vi "副屏设置.vi"() -> ()   [LabVIEW 2016, in "副屏.lvlib"]
uses:
  <vilib>/Utility/config.llb/NI_LVConfig.lvlib
panel:
  in  "藻密度":bool=TRUE caption="氨氮禁用"
  in  "叶绿素a":bool=TRUE caption="氨氮禁用"
  in  "启用副屏":bool=TRUE caption="氨氮禁用"
  in  "关闭":bool
  in  "底部状态栏显示信息":string="一体化微型水质监测系统"
  in  "流速":bool caption="氨氮禁用"
  in  "瞬时流量":bool caption="氨氮禁用"
  in  "湿度":bool=TRUE caption="氨氮禁用"
  in  "水位":bool caption="氨氮禁用"
  in  "室温":bool=TRUE caption="氨氮禁用"
  in  "CODCr":bool caption="氨氮禁用"
  in  "CODMn":bool caption="氨氮禁用"
  in  "总氮":bool caption="氨氮禁用"
  in  "总磷":bool caption="氨氮禁用"
  in  "氨氮":bool caption="氨氮禁用"
  in  "Turb":bool caption="氨氮禁用"
  in  "Cond":bool caption="氨氮禁用"
  in  "DO":bool caption="氨氮禁用"
  in  "pH":bool caption="氨氮禁用"
  in  "水温":bool caption="氨氮禁用"
  # "副屏显示信息设置"
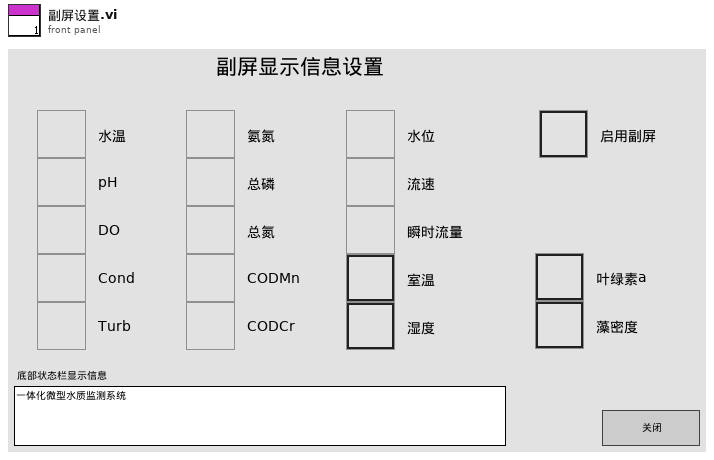
[diagram p1: front panel]
types:
  T1 = typedef "NI_LVConfig.lvlib/Config Data RefNum.ctl" = refnum<k1>
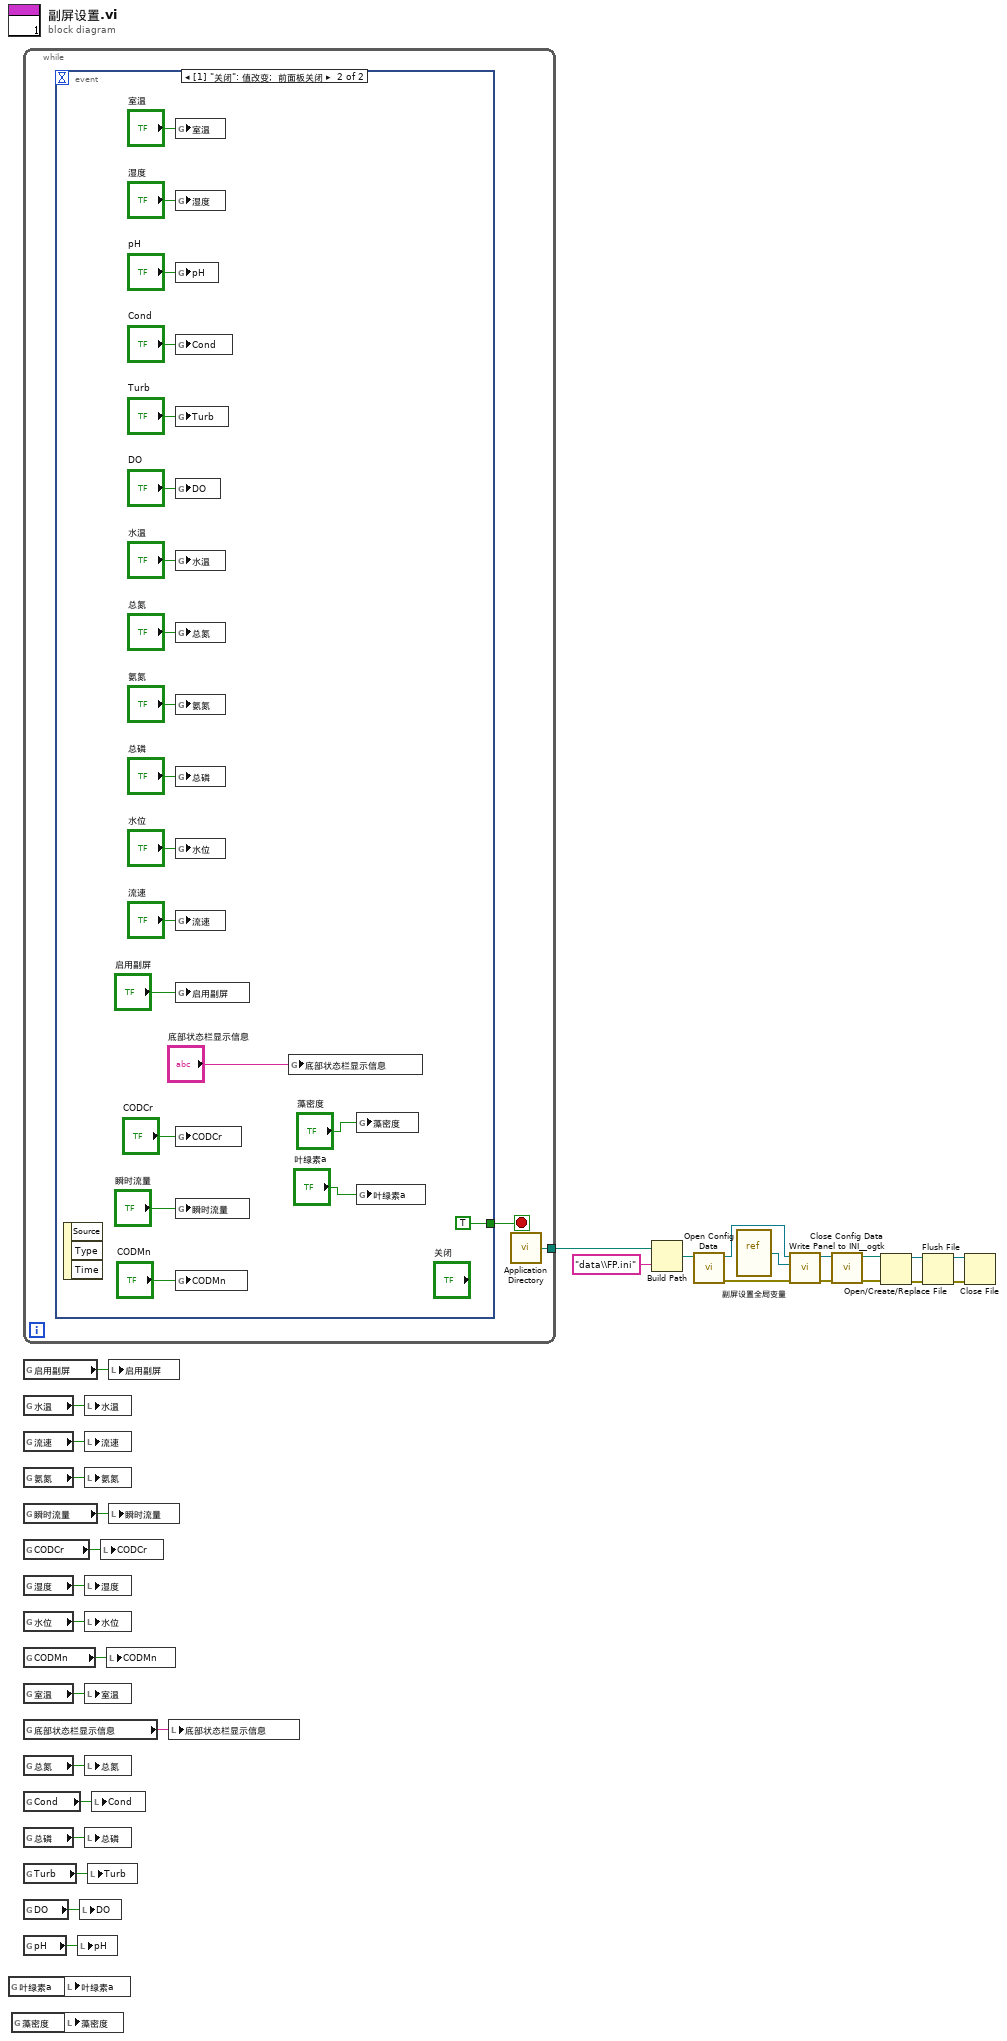
[diagram p0: block diagram]
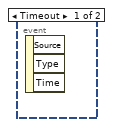
[diagram p2: hidden frame]
diagram:
  n1 = global read "副屏设置全局变量.vi" "叶绿素a"() -> (w7:bool)
  n2 = global read "副屏设置全局变量.vi" "藻密度"() -> (w8:bool)
  n3 = while {
    tunnel: [w34] -> w10
    stop <- w35 stop-if-true
    n4 = event shown="[1] \"关闭\": 值改变;  前面板关闭" {
      selector: _ -> [_ _]
      dyn-events: _ -> [_ _]
      timeout: _ -> [_ _]
      tunnel: [_ TRUE] -> w35
      event Timeout {
        n5 = event-data() -> ()  [unwired: 1 in, 3 out]
      }
      event "关闭": Value Change; Panel Close {
        n6 = event-data() -> ()  [unwired: 1 in, 3 out]
        n7 = global write "副屏设置全局变量.vi" "室温"("室温") -> ()
        n8 = global write "副屏设置全局变量.vi" "湿度"("湿度") -> ()
        n9 = global write "副屏设置全局变量.vi" "pH"("pH") -> ()
        n10 = global write "副屏设置全局变量.vi" "Cond"("Cond") -> ()
        n11 = global write "副屏设置全局变量.vi" "Turb"("Turb") -> ()
        n12 = global write "副屏设置全局变量.vi" "DO"("DO") -> ()
        n13 = global write "副屏设置全局变量.vi" "水温"("水温") -> ()
        n14 = global write "副屏设置全局变量.vi" "总氮"("总氮") -> ()
        n15 = global write "副屏设置全局变量.vi" "氨氮"("氨氮") -> ()
        n16 = global write "副屏设置全局变量.vi" "总磷"("总磷") -> ()
        n17 = global write "副屏设置全局变量.vi" "水位"("水位") -> ()
        n18 = global write "副屏设置全局变量.vi" "流速"("流速") -> ()
        n19 = global write "副屏设置全局变量.vi" "启用副屏"("启用副屏") -> ()
        n20 = global write "副屏设置全局变量.vi" "CODCr"("CODCr") -> ()
        n21 = global write "副屏设置全局变量.vi" "瞬时流量"("瞬时流量") -> ()
        n22 = global write "副屏设置全局变量.vi" "CODMn"("CODMn") -> ()
        n23 = global write "副屏设置全局变量.vi" "底部状态栏显示信息"("底部状态栏显示信息") -> ()
        n24 = global write "副屏设置全局变量.vi" "藻密度"("藻密度") -> ()
        n25 = global write "副屏设置全局变量.vi" "叶绿素a"("叶绿素a") -> ()
      }
    }
    n26 = call <vilib>:"Application Directory.vi"() -> ("Application Directory"=w34:path)
  }
  n27 = global read "副屏设置全局变量.vi" "启用副屏"() -> (w9:bool)
  n28 = global read "副屏设置全局变量.vi" "水温"() -> (w33:bool)
  n29 = global read "副屏设置全局变量.vi" "流速"() -> (w27:bool)
  n30 = global read "副屏设置全局变量.vi" "氨氮"() -> (w32:bool)
  n31 = global read "副屏设置全局变量.vi" "瞬时流量"() -> (w25:bool)
  n32 = global read "副屏设置全局变量.vi" "CODCr"() -> (w31:bool)
  n33 = global read "副屏设置全局变量.vi" "湿度"() -> (w24:bool)
  n34 = global read "副屏设置全局变量.vi" "水位"() -> (w30:bool)
  n35 = global read "副屏设置全局变量.vi" "CODMn"() -> (w29:bool)
  n36 = global read "副屏设置全局变量.vi" "室温"() -> (w21:bool)
  n37 = global read "副屏设置全局变量.vi" "底部状态栏显示信息"() -> (w28:string)
  n38 = global read "副屏设置全局变量.vi" "总氮"() -> (w22:bool)
  n39 = global read "副屏设置全局变量.vi" "Cond"() -> (w26:bool)
  n40 = global read "副屏设置全局变量.vi" "总磷"() -> (w19:bool)
  n41 = global read "副屏设置全局变量.vi" "Turb"() -> (w20:bool)
  n42 = global read "副屏设置全局变量.vi" "DO"() -> (w23:bool)
  n43 = global read "副屏设置全局变量.vi" "pH"() -> (w18:bool)
  n44 = local write "叶绿素a"(w7) -> ()
  n45 = local write "藻密度"(w8) -> ()
  n46 = local write "pH"(w18) -> ()
  n47 = local write "DO"(w23) -> ()
  n48 = local write "水温"(w33) -> ()
  n49 = local write "流速"(w27) -> ()
  n50 = local write "氨氮"(w32) -> ()
  n51 = local write "湿度"(w24) -> ()
  n52 = local write "水位"(w30) -> ()
  n53 = local write "室温"(w21) -> ()
  n54 = local write "总氮"(w22) -> ()
  n55 = local write "总磷"(w19) -> ()
  n56 = local write "Turb"(w20) -> ()
  n57 = local write "Cond"(w26) -> ()
  n58 = local write "CODCr"(w31) -> ()
  n59 = local write "CODMn"(w29) -> ()
  n60 = local write "启用副屏"(w9) -> ()
  n61 = local write "瞬时流量"(w25) -> ()
  n62 = local write "底部状态栏显示信息"(w28) -> ()
  n63 = Build Path(base path=w10, name or relative path="data\\FP.ini" ("名称或相对路径")) -> (appended path=w12:path)
  n64 = call <vilib>:"Open Config Data.vi"("configuration file path"=w12) -> ("error out"=w16:errorcluster, "refnum"=w13:T1)  [unwired: 8 in, 1 out]
  n65 = vi-ref "副屏设置全局变量.vi"() -> (w14:refnum<vi>)
  n66 = call <userlib>:"Write Panel to INI__ogtk.vi"("error in (no error)"=w16, "VI ref"=w14, "refnum"=w13) -> ("error out"=w17:errorcluster, "refnum out"=w15:T1)  [unwired: 7 in]
  n67 = call <vilib>:"Close Config Data.vi"("error in (no error)"=w17, "refnum"=w15) -> ("error out"=w1:errorcluster, "file path"=w2:path)  [unwired: 8 in]
  n68 = Open/Create/Replace File(file path (use dialog)=w2, error in=w1) -> (refnum out=w5:refnum<file>, error out=w6:errorcluster)  [unwired: 4 in, 1 out]
  n69 = Flush File(refnum=w5, error in=w6) -> (refnum out=w4:refnum<file>, error out=w3:errorcluster)
  n70 = Close File(refnum=w4, error in=w3) -> ()  [unwired: 2 out]
